vi "Convert Signal to Banks.vi"(8 "error in":errorcluster, 11 "SL_SC in":refnum<class "SL_SC.lvclass">) -> (0 "error out":errorcluster, 3 "SL_SC out":refnum<class "SL_SC.lvclass">)   [LabVIEW 2019, in "SL_SC.lvlib" / "SL_SC.lvclass"]
uses:
  Library/SL_SC.lvclass
  C:/Users/Public/Documents/Development/builds/Instruments/DIG_IO.lvlibp/Library/DIG_IO.lvclass
  builds/Instruments/DIG_IO.lvlibp/Accessors/Read BankDefs.vi
  builds/Instruments/DIG_IO.lvlibp/Accessors/Read Digital.vi
  builds/Instruments/DIG_IO.lvlibp/Accessors/Write Banks.vi
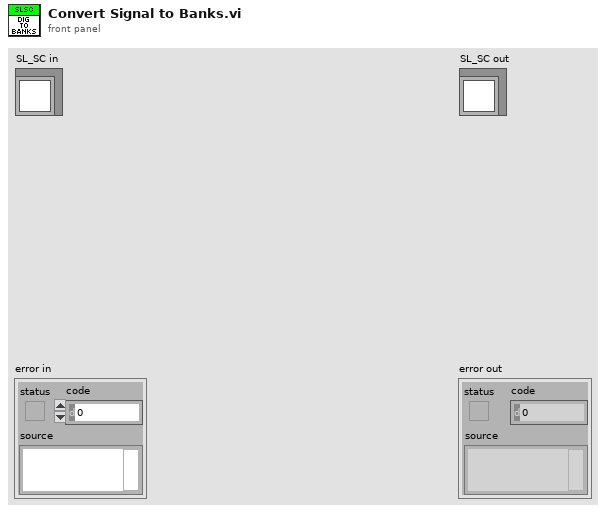
[diagram p1: front panel]
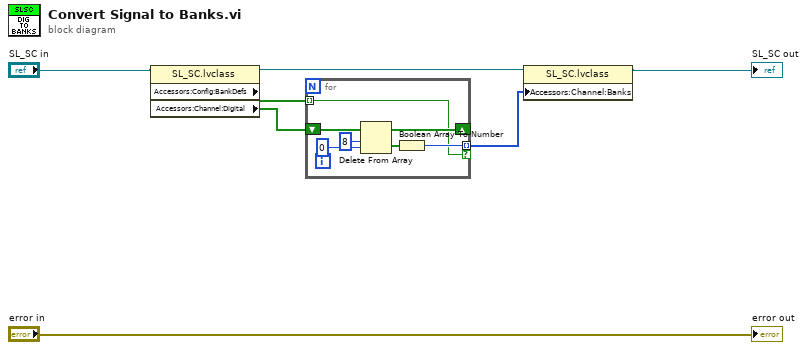
[diagram p0: block diagram]
diagram:
  n1 = property class="SL_SC.lvclass"(reference="SL_SC in") -> (reference out=w4:refnum<class "SL_SC.lvclass">, "Accessors:Config:BankDefs"=w6:bool[], "Accessors:Channel:Digital"=w5:bool[])  [unwired: 1 in, 1 out]
  n2 = for {
    tunnel: w6 -> [w8] mode=indexing
    shift-right: [w11] -> _
    shift-left: w5 -> [w14]
    tunnel: [w9] -> w7 mode=indexing if=w8
    n3 = Delete From Array(array=w14, length=8, index=0) -> (deleted portion=w10:bool[], array with subset deleted=w11:bool[])
    n4 = Boolean Array To Number(Boolean array=w10) -> (number=w9:u8)
  }
  n5 = property class="SL_SC.lvclass"(reference=w4, "Accessors:Channel:Banks"=w7) -> (reference out=→"SL_SC out":refnum<class "SL_SC.lvclass">)  [unwired: 1 in, 1 out]
  "error out" <- "error in"
